vi "Write Number of channels.vi"(8 "error in (no error)":errorcluster, 10 "Number of channels":i32=2, 11 "Red Pitaya Digitizer in":refnum<class "Red Pitaya Digitizer.lvclass">) -> (0 "error out":errorcluster, 3 "Red Pitaya Digitizer out":refnum<class "Red Pitaya Digitizer.lvclass">)   [LabVIEW 2020, in "Red Pitaya Digitizer.lvclass"]
uses:
  Red Pitaya Digitizer.lvclass
  Red Pitaya Digitizer.lvclass/Red Pitaya Digitizer.ctl
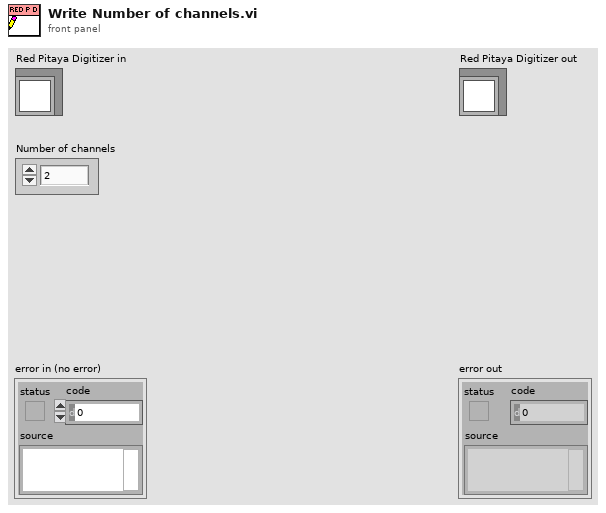
[diagram p1: front panel]
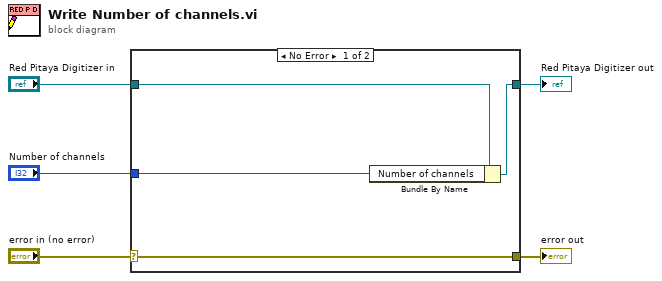
[diagram p0: block diagram]
diagram:
  n1 = case shown="No Error" "error in (no error)" {
    selector: "error in (no error)" -> [w9 w10]
    tunnel: [w9 w10] -> w4
    tunnel: [w7 w11] -> w2
    tunnel: "Red Pitaya Digitizer in" -> [w8 w11]
    tunnel: "Number of channels" -> [w6 _]
    frame No Error {
      n2 = Bundle By Name(cluster=w8, "Number of channels"=w6) -> (w7:refnum<class "Red Pitaya Digitizer.lvclass">)
    }
    frame Error {
    }
  }
  "error out" <- w4
  "Red Pitaya Digitizer out" <- w2
